vi "Update Status.vi"(10 "Result":T1, 11 "Result Model in":refnum<class "Result Model.lvclass">) -> ()   [LabVIEW 2020, in "Result Model.lvclass"]
uses:
  Result Model.lvclass
  Core/Result/Result.ctl
  Core/Result/Status.ctl
  Core/Result/Type.ctl
  Result Model.lvclass/Result Model.ctl
  <vilib>/Utility/miscctls.llb/LVMapReplaceAction.ctl
  Core/Result/Result.lvlib
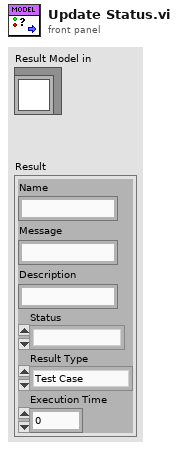
[diagram p1: front panel]
types:
  T1 = typedef "Result.lvlib/Result.ctl" = cluster{"Name":string, "Message":string, "Description":string, "Status":T2, "Result Type":T3, "Execution Time":dbl}
  T2 = typedef "Result.lvlib/Status.ctl" = enum16{"", "Passed", "Failed", "Error", "Skipped", "Setup Error", "Broken", "Teardown Error"}
  T3 = typedef "Result.lvlib/Type.ctl" = enum16{"Test Case", "Test Suite", "Test Run", "Pass", "Fail", "Skip", "Pass if", "Fail if", "Pass if Error", "Fail if Error", "Pass if Equal", "Fail if Equal"}
  T4 = typedef "LVMapReplaceAction.ctl" = enum32{"Modify Entry only if found", "Add or Modify Entry", "Delete Entry"}
  T5 = cluster{"Result Type":T3, "Status":T2, "Message":string, "Description":string}
  T6 = typedef "Result Model.lvclass/Model State.ctl" = cluster{"Run Queue":set{string}, "Test Statuses":map{string, T2}, "Execution Time":map{string, dbl}, "Assertions":map{string, cluster{"Result Type":T3, "Status":T2, "Message":string, "Description":string}[]}}
  T7 = map{string, cluster{"Result Type":T3, "Status":T2, "Message":string, "Description":string}[]}
  T8 = cluster{"Result Type":T3, "Status":T2, "Message":string, "Description":string}[]
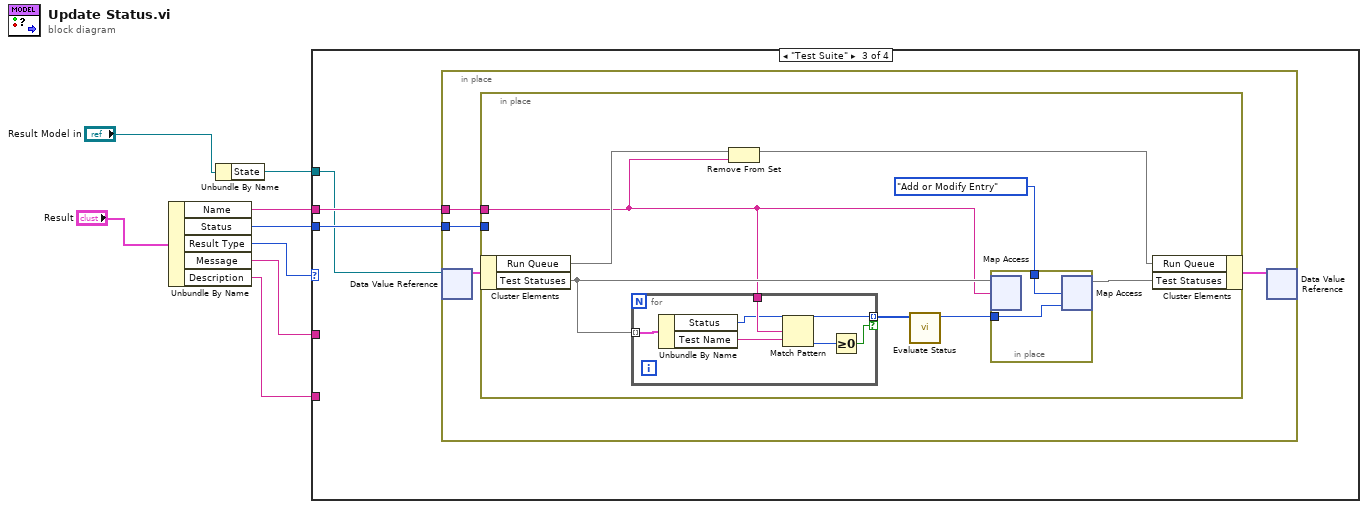
[diagram p0: block diagram]
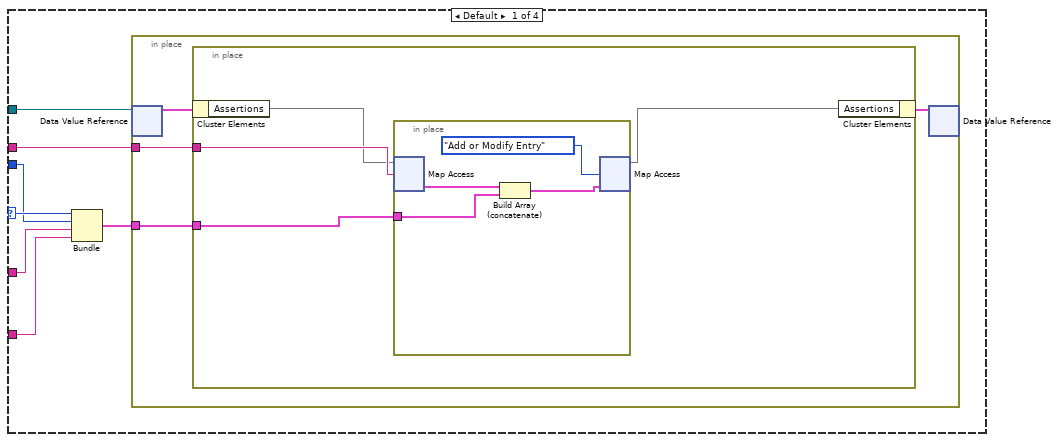
[diagram p2: hidden frame]
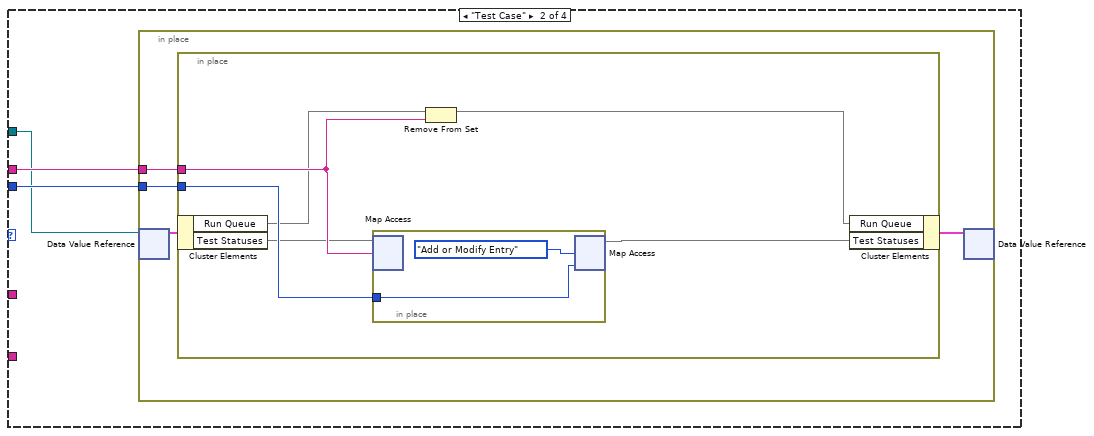
[diagram p3: hidden frame]
diagram:
  n1 = Unbundle By Name("Result") -> ("Name"=w8:string, "Status"=w7:T2, "Result Type"=w5:T3, "Message"=w4:string, "Description"=w3:string)
  n2 = Unbundle By Name("Result Model in") -> ("State"=w2:refnum<data-value>)
  n3 = case shown="\"Test Suite\"" w5 {
    selector: w5 -> [w11 _ _ _]
    tunnel: w8 -> [w12 w30 w45 _]
    tunnel: w7 -> [w10 w29 w44 _]
    tunnel: w4 -> [w14 _ _ _]
    tunnel: w3 -> [w13 _ _ _]
    tunnel: w2 -> [w9 w28 w43 _]
    frame Default {
      n4 = Bundle("Result Type"=w11, "Status"=w10, "Message"=w14, "Description"=w13) -> (w15:T5)  [unwired: 1 in]
      n5 = in-place {
        in-place-border: w15 -> [w19]
        in-place-border: w12 -> [w18]
        n6 = in-place-dvr #1(w9) -> (w17:T6)  [unwired: 1 out]
        n7 = in-place {
          in-place-border: w19 -> [w23]
          in-place-border: w18 -> [w22]
          n8 = in-place-cluster #2(w17) -> ("Assertions"=w21:T7)
          n9 = in-place {
            in-place-border: w23 -> [w25]
            n10 = in-place-map #3(w21, w22) -> (w27:T8)  [unwired: 1 in, 1 out]
            n11 = Build Array (concatenate)(w27, w25) -> (w26:T8)
            n12 = in-place-map #3(w26, LVMapReplaceAction."Add or Modify Entry" ("action")) -> (w20:T7)  [unwired: 2 out]
          }
          n13 = in-place-cluster #2("Assertions"=w20) -> (w16:T6)
        }
        n14 = in-place-dvr #1(w16) -> ()  [unwired: 2 out]
      }
    }
    frame "Test Case" {
      n15 = in-place {
        in-place-border: w30 -> [w34]
        in-place-border: w29 -> [w33]
        n16 = in-place-dvr #4(w28) -> (w32:T6)  [unwired: 1 out]
        n17 = in-place {
          in-place-border: w34 -> [w40]
          in-place-border: w33 -> [w39]
          n18 = in-place-cluster #5(w32) -> ("Run Queue"=w38:set{string}, "Test Statuses"=w37:map{string, T2})
          n19 = in-place {
            in-place-border: w39 -> [w41]
            n20 = in-place-map #6(w37, w40) -> ()  [unwired: 1 in, 2 out]
            n21 = in-place-map #6(w41, LVMapReplaceAction."Add or Modify Entry" ("action")) -> (w35:map{string, T2})  [unwired: 2 out]
          }
          n22 = Remove From Set(10:w40, 11:w38) -> (3:w36:set{string})  [unwired: 1 out]
          n23 = in-place-cluster #5("Run Queue"=w36, "Test Statuses"=w35) -> (w31:T6)
        }
        n24 = in-place-dvr #4(w31) -> ()  [unwired: 2 out]
      }
    }
    frame "Test Suite" {
      n25 = in-place {
        in-place-border: w45 -> [w49]
        in-place-border: w44 -> [w48]
        n26 = in-place-dvr #7(w43) -> (w47:T6)  [unwired: 1 out]
        n27 = in-place {
          in-place-border: w49 -> [w52]
          in-place-border: w48 -> [_]
          n28 = in-place-cluster #8(w47) -> ("Run Queue"=w57:set{string}, "Test Statuses"=w54:map{string, T2})
          n29 = for {
            tunnel: w54 -> [w63] mode=indexing
            tunnel: w52 -> [w61]
            tunnel: [w59] -> w51 mode=indexing if=w58
            n30 = Unbundle By Name(w63) -> ("Status"=w59:T2, "Test Name"=w62:string)
            n31 = Match Pattern(string=w62, regular expression=w61) -> (offset past match=w60:i32)  [unwired: 1 in, 3 out]
            n32 = Greater Or Equal To 0?(x=w60) -> (x >= 0?=w58:bool)
          }
          n33 = Remove From Set(10:w52, 11:w57) -> (3:w56:set{string})  [unwired: 1 out]
          n34 = call "Evaluate Status.vi"("Statuses"=w51) -> ("Status"=w50:T2)  [unwired: 10 in]
          n35 = in-place {
            in-place-border: LVMapReplaceAction."Add or Modify Entry" ("action") -> [w65]
            in-place-border: w50 -> [w64]
            n36 = in-place-map #9(w54, w52) -> ()  [unwired: 1 in, 2 out]
            n37 = in-place-map #9(w64, w65) -> (w55:map{string, T2})  [unwired: 2 out]
          }
          n38 = in-place-cluster #8("Run Queue"=w56, "Test Statuses"=w55) -> (w46:T6)
        }
        n39 = in-place-dvr #7(w46) -> ()  [unwired: 2 out]
      }
    }
    frame "Test Run" {
    }
  }
